vi "DequeueData.vi"(8 "error in (no error)":errorcluster, 9 "timeout in ms (-1)":i32, 10 "DataIn":T1={"t0"=timestamp(0 s since 1904-01-01), "dt"=1.0, "attributes"=variant, "Y_ref"=refnum} {"dt" format="%0.6f"; "t0" format="%<%X\n%x>T"}, 11 "queue in":refnum<queue>) -> (0 "error out":errorcluster, 1 "timed out?":bool, 2 "Data Out":T1={"t0"=timestamp(0 s since 1904-01-01), "dt"=1.0, "attributes"=variant, "Y_ref"=refnum} {"dt" format="%0.6f"; "t0" format="%<%X\n%x>T"}, 3 "queue out":refnum<queue>, 5 "Y":dbl[][](array[numeric]))   [LabVIEW 2018, in "AnalysisPlugins.lvlib" / "FitterBase.lvclass"]
uses:
  FitterBase.lvclass
  AnalysisPluginBaseClass/Typedefs/SampleDataInput.ctl
  Typedefs/Wvfrm_ref.ctl
  AnalysisPluginBaseClass/AnalysisPluginsBase.lvclass
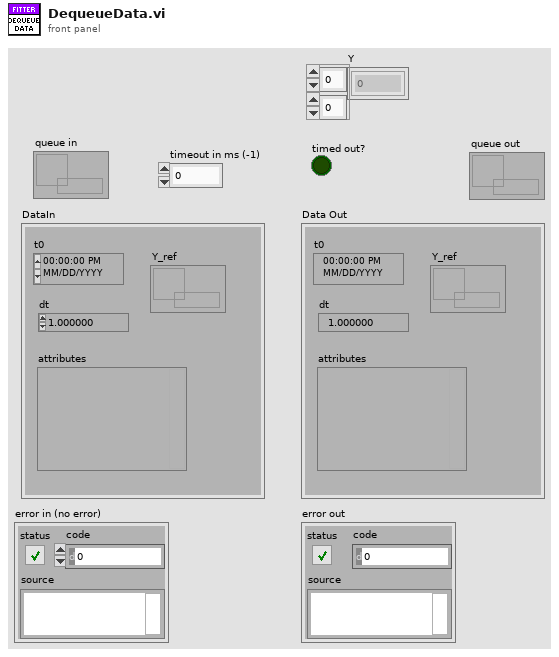
[diagram p1: front panel]
types:
  T1 = typedef "AnalysisPlugins.lvlib/FitterBase.lvclass/Wvfrm_ref.ctl" = cluster{"t0":timestamp, "dt":dbl, "attributes":variant, "Y_ref":refnum<data-value>}
  T2 = typedef "AnalysisPlugins.lvlib/AnalysisPluginsBase.lvclass/SampleDataInput.ctl" = waveform(dbl)[]
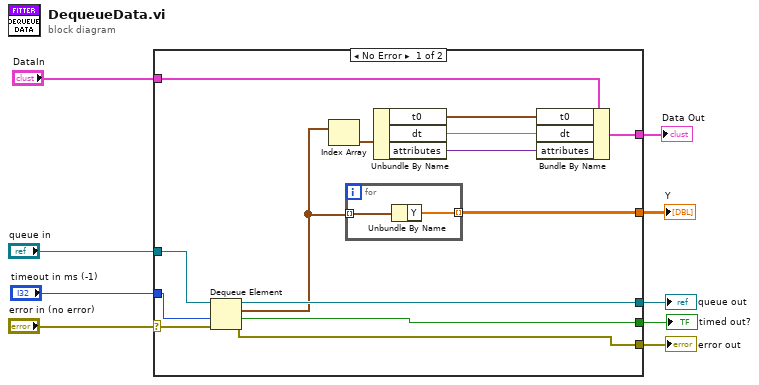
[diagram p0: block diagram]
diagram:
  n1 = case shown="No Error" "error in (no error)" {
    selector: "error in (no error)" -> [w17 w26]
    tunnel: [w23 w27] -> w9
    tunnel: [w22 _] -> w8
    tunnel: "timeout in ms (-1)" -> [w16 _]
    tunnel: "queue in" -> [w15 w27]
    tunnel: "DataIn" -> [w13 w28]
    tunnel: [w12 w28] -> w3
    tunnel: [w11 w26] -> w2
    tunnel: [w10 _] -> w1
    frame No Error {
      n2 = Dequeue Element(queue=w15, timeout in ms (-1)=w16, error in (no error)=w17) -> (queue out=w23:refnum<queue>, element=w14:T2, timed out?=w22:bool, error out=w11:errorcluster)
      n3 = Index Array(array=w14) -> (element=w21:waveform(dbl))  [unwired: 1 in]
      n4 = for {
        tunnel: w14 -> [w25] mode=indexing
        tunnel: [w24] -> w10 mode=indexing
        n5 = Unbundle By Name(w25) -> ("Y"=w24:dbl[])
      }
      n6 = Unbundle By Name(w21) -> ("t0"=w20:timestamp, "dt"=w19:dbl, "attributes"=w18:variant)
      n7 = Bundle By Name(cluster=w13, "t0"=w20, "dt"=w19, "attributes"=w18) -> (w12:T1)
    }
    frame Error {
    }
  }
  "error out" <- w2
  "timed out?" <- w8
  "queue out" <- w9
  "Data Out" <- w3
  "Y" <- w1
